vi "LATEX.vi"(0 "NO SP":string, 1 "TO":string, 2 "SENT BY":string, 3 "GOODS":string[][](table), 4 "PACKED BY":string, 9 "FILEPATH":path, 11 "Filename":string) -> (14 "string":string)   [LabVIEW 2018]
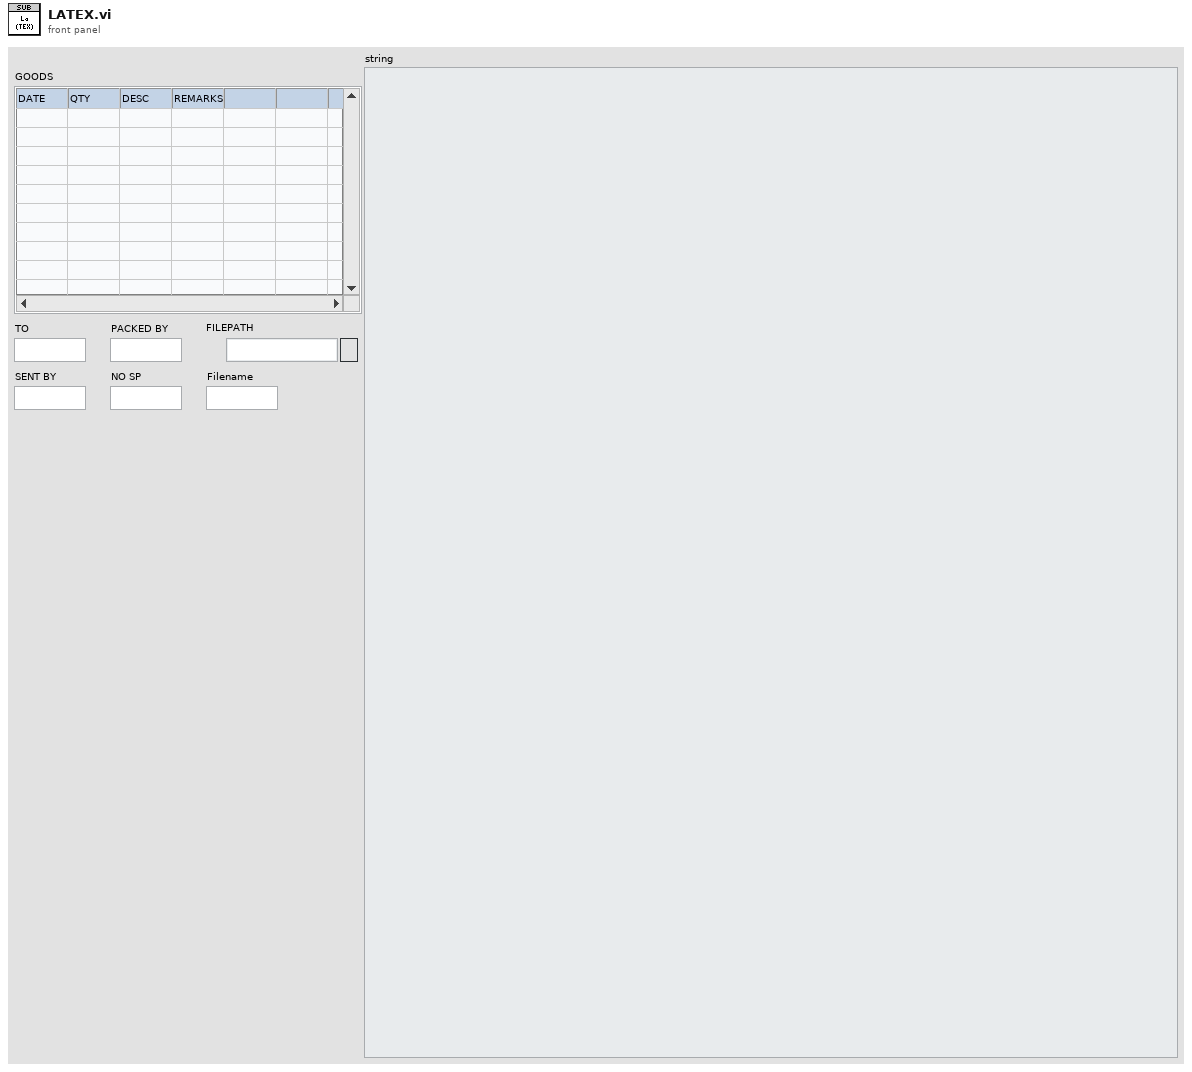
[diagram p1: front panel]
types:
  T1 = enum16{"open", "replace", "create", "open or create", "replace or create", "replace or create with confirmation"}
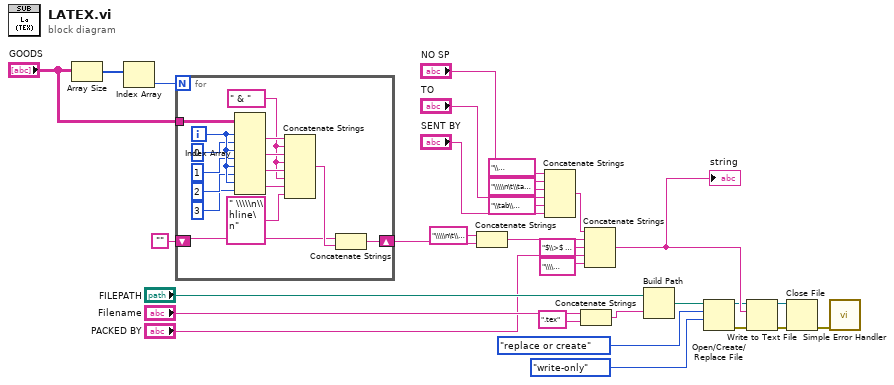
[diagram p0: block diagram]
diagram:
  n1 = Array Size(array="GOODS") -> (size(s)=w30:i32[])
  n2 = Index Array(array=w30) -> (element=w29:i32)  [unwired: 1 in]
  n3 = for {
    N: w29 -> [_]
    tunnel: "GOODS" -> [w45]
    shift-right: [w32] -> w26
    shift-left: "" -> [w31]
    i -> [w44]
    w36 = " & "
    n4 = Index Array(array=w45, index (row) #1=w44, index (col) #1=0 ("disabled index (col)"), index (row) #2=w44, index (col) #2=1 ("disabled index (col)"), index (row) #3=w44, index (col) #3=2 ("disabled index (col)"), index (row) #4=w44, index (col) #4=3 ("disabled index (col)")) -> (element #1=w39:string, element #2=w38:string, element #3=w37:string, element #4=w35:string)
    n5 = Concatenate Strings(w39, w36, w38, w36, w37, w36, w35, " \\\\\n\\hline\n" ("string")) -> (w33:string)
    n6 = Concatenate Strings(w31, w33) -> (w32:string)
  }
  n7 = Concatenate Strings("\\\\\n\t\\qquad\\quad Sent by:\n}\n\\lfoot{\n\t\\qquad\\quad GMF/A-11\\tab\\qquad\\qquad\\qquad\\qquad\\qquad\\qquad\\qquad\\qquad\\qquad\\qquad\\qquad\\thepage\\ of \\pageref{LastPage}\n}\n\n\\begin{document}\n\t$\\>$\\\\\n\t$\\>$\\\\\n\t$\\>$\\\\\n\t$\\>$\\\\\n\t\\begin{center}\n\t\\begin{longtable}{|P{.10\\textwidth}|P{.09\\textwidth}|V{.38\\textwidth}|V{.20\\textwidth}|}\n\t\\hline\n\t\\parbox[P]{.10\\textwidth}{\\centering\\textbf{\\underline{Tanggal}}\\\\Date} &\n\t\\parbox[P]{.09\\textwidth}{\\centering\\textbf{\\underline{Banyaknya}}\\\\Quantity} &\n\t\\parbox[V]{.38\\textwidth}{\\centering\\textbf{\\underline{Macam dari barang-barang}}\\\\Description of goods} &\n\t\\parbox[V]{.20\\textwidth}{\\centering\\textbf{\\underline{Keterangan}}\\\\Remarks} \\\\\n\t\\hline\n\t\\endhead\n" ("string"), w26) -> (w20:string)
  n8 = Concatenate Strings("\\documentclass{article}\n\\usepackage{tabto}\n\\usepackage{geometry}\n\\geometry{\n \ta4paper,\n\tincludefoot,\n\tleft=5mm,\n\tright=5mm,\n \ttotal={170mm,257mm},\n \ttop=20mm,\n }\n\\usepackage{longtable}\n\\usepackage{lipsum}\n\\usepackage{graphicx}\n\\usepackage{fancyhdr}\n\\usepackage{needspace}\n\\usepackage{lastpage}\n\\usepackage{array}\n\\newcolumntype{P}[1]{>{\\centering\\arraybackslash}m{#1}}\n\\newcolumntype{V}[1]{>{\\raggedright\\arraybackslash}m{#1}}\n\\pagestyle{fancy}\n\\fancyfoot{}\n\\renewcommand{\\headrulewidth}{0pt}\n\\renewcommand{\\arraystretch}{2.0}\n\\addtolength{\\textheight}{-80.0pt}\n\\lhead{\n\t\\qquad\\quad\\includegraphics[width=200px]{./images/gmf}\n\t\\tab\\qquad\\qquad\\qquad\\qquad\\qquad\\qquad\\quad NO. SP. " ("string"), "NO SP", "\\\\\n\t\\tab\\qquad\\qquad\\qquad\\qquad\\qquad\\qquad\\quad\\textbf{\\underline{SURAT PENGIRIMAN}}\\\\\n\t\\qquad\\quad\\textbf{\\underline{Kepada}}\\quad\\quad\\quad\\quad: " ("string"), "TO", "\\tab\\qquad\\qquad\\qquad\\qquad\\qquad\\qquad\\quad Shipping Document\\\\\n\t\\qquad\\quad To:\\\\\n\t\\qquad\\quad\\textbf{\\underline{Dikirim oleh}}$\\>$$\\>$\\quad: " ("string"), "SENT BY") -> (w21:string)
  n9 = Concatenate Strings("Filename", ".tex" ("string")) -> (w11:string)
  n10 = Concatenate Strings(w21, w20, "$\\>$ & $\\>$ &\\raggedright\\parbox[V]{.38\\textwidth}{\\textbf{\\underline{Dikirim oleh}}: " ("string"), "PACKED BY", "\\\\Packed by} & $\\>$ \\\\\n\t\\hline\n\t\\end{longtable}\n\t\\end{center}\n\\Needspace{5\\baselineskip}\n\\quad $\\>$ \\textbf{\\underline{Tanda tangan penerima}}:\\tab\\qquad\\qquad\\qquad\\qquad\\qquad\\qquad\\qquad\\qquad Original : Shipper\\\\\n\\tab\\qquad\\quad Sign received\\tab\\qquad\\qquad\\qquad\\qquad\\qquad\\qquad\\qquad\\qquad Copy 1 : Receiver\\\\\n$\\>$\\tab\\tab\\tab\\qquad\\qquad\\qquad\\qquad\\qquad\\qquad\\qquad\\qquad Copy 2 : File\\\\\n\\tab\\qquad\\quad\\textbf{\\underline{Tgl}}:\\\\\n\\tab\\qquad\\quad Date\n\\end{document}" ("string")) -> (w15:string)
  "string" <- w15
  n11 = Build Path(base path="FILEPATH", name or relative path=w11) -> (appended path=w8:path)
  n12 = Open/Create/Replace File(file path (use dialog)=w8, operation (0:open)=T1."replace or create", access (0:read/write)=enum16{"read/write", "read-only", "write-only"}."write-only") -> (refnum out=w13:refnum<file>, error out=w14:errorcluster)  [unwired: 3 in, 1 out]
  n13 = Write to Text File(file (use dialog)=w13, text=w15, error in=w14) -> (refnum out=w16:refnum<file>, error out=w17:errorcluster)  [unwired: 1 in, 1 out]
  n14 = Close File(refnum=w16, error in=w17) -> (error out=w1:errorcluster)  [unwired: 1 out]
  n15 = call <vilib>:"Simple Error Handler.vi"("error in (no error)"=w1) -> ()  [unwired: 4 in, 5 out]
